vi "OE2011&OE2021_Configure Demodulator Reference.vi"(7 "OE2012&OE2022_Configure Demodulator Ref":T1={"Demodulator"=1, "Ref. Source"=0, "Arb Frequency"=1000.0, "Ref. Harmonic"=1, "Ref. Phase(degree)"=0.0, "Instrument Mode "=10, "A"=1000, "F1"=0, "B"=1000, "F2"=0} {"F2" items=["OSC1", "OSC2", "Demod MF1", "Demod MF2", "Demod MF3", "Demod MF4", "Demod MF5", "Demod MF6", "Demod MF7", "Demod MF8"]; "B" min=-10000 max=10000; "F1" items=["OSC1", "OSC2", "Demod MF1", "Demod MF2", "Demod MF3", "Demod MF4", "Demod MF5", "Demod MF6", "Demod MF7", "Demod MF8"]; "A" min=-10000 max=10000; "Instrument Mode" items=["OE2012"=10, "OE2022"=11]; "Ref. Phase(degree)" min=-180.0 max=180.0 format="%#.2g"; "Ref. Harmonic" min=1 max=32767; "Arb Frequency" min=1e-06 max=1002000.0 format="%#.3f"; "Ref. Source" items=["OSC1", "OSC2", "ManualFrequency", "FreqComb1", "FreqComb2", "FreqComb3", "FreqComb4"]; "Demodulator" items=["Demod1"=1, "Demod2"=2, "Demod3"=3, "Demod4"=4, "Demod5"=5, "Demod6"=6, "Demod7"=7, "Demod8"=8]}, 8 "Error in (no error)":errorcluster caption="error out（no error）", 9 "Remote Mode":u16(ring)=1 items=["USB", "RS232", "GPIB", "Ethernet"], 10 "Connection ID in":refnum<k5>, 11 "VISA resource name":refnum<visa-resource-name>) -> (0 "Error out":errorcluster caption="error out", 1 "Output String":string, 2 "Connection ID out":refnum<k5>, 3 "VISA resource  out":refnum<visa-resource-name>)   [LabVIEW 2011]
panel:
  out "Demod Channel":string
  # "E = A * Osc + B * Freq"
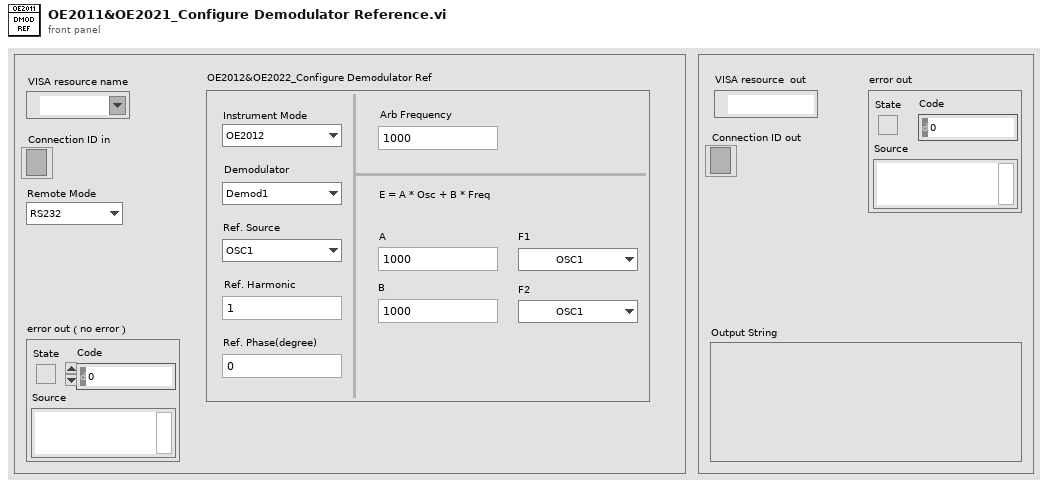
[diagram p1: front panel]
types:
  T1 = cluster{"Demodulator":u16, "Ref. Source":u16, "Arb Frequency":dbl, "Ref. Harmonic":u16, "Ref. Phase(degree)":dbl, "Instrument Mode ":u16, "A":i16, "F1":u16, "B":i16, "F2":u16}
  T2 = enum16{"ISRC", "IGND", "ICPL", "ILIN", "PHAS", "FMOD", "RSLP", "FREQ", "SWPT", "SLLM", "SULM", "SSLL", "SSLG", "STLM", "SWRM", "IRNG", "SENS", "RMOD", "OFLT", "OFSL", "SYNC", "DMOD", "HARM", "DARB", "SWVT", "SLVL", "SVLL", "SVUL", "SVSL", "SVSG", "SVTM", "SVRM", "RALL", "SNAP", "OUTP", "OAUX", "COUT", "CAUX", "COFP", "CEXP", "FPOP", "OEXP", "*IDN", "*RST", "OVLD", "INOV", "GNOV", "*PLL", "SSET", "RSET", "AGAN", "APHS", "ARSV", "ASCL", "EQCD", "EQCS", "SPED", "SRAT", "SLEN", "SSLE", "STRG", "SPRM", "STRD", "PAUS", "REST", "SPTS", "TRCA", "TEMP", "RSTU", "IHNZ", "DEQU", "SADD", "ARNG", "CSPE", "ISRCD", "IGNDD", "ICPLD", "ILIND", "PHASD", "FMODD", "RSLPD", "FREQD", "SWPTD", "SLLMD", "SULMD", "SSLLD", "SSLGD", "STLMD", "SWRMD", "SENSD", "RMODD", "OFLTD", "OFSLD", "SYNCD", "HARMD", "EQCDD", "EQCSD", "SNAPD", "OUTPD", "SWVTD", "SLVLD", "SVLLD", "SVULD", "SVSLD", "SVSGD", "SVTMD", "SVRMD", "SVDCD", "ARSVD", "AGAND", "APHSD", "ASCLD", "FPOPD", "CAUXD", "OEXPD", "SPEDD", "SRATD", "SLEND", "SSLED", "STRGD", "SPRMD", "STRDD", "PAUSD", "RESTD", "SPTSD", "TRCAD", "*IDND", "*RSTD", "INOVD", "GNOVD", "*PLLD", "SSETD", "RSETD", "RALLD"}
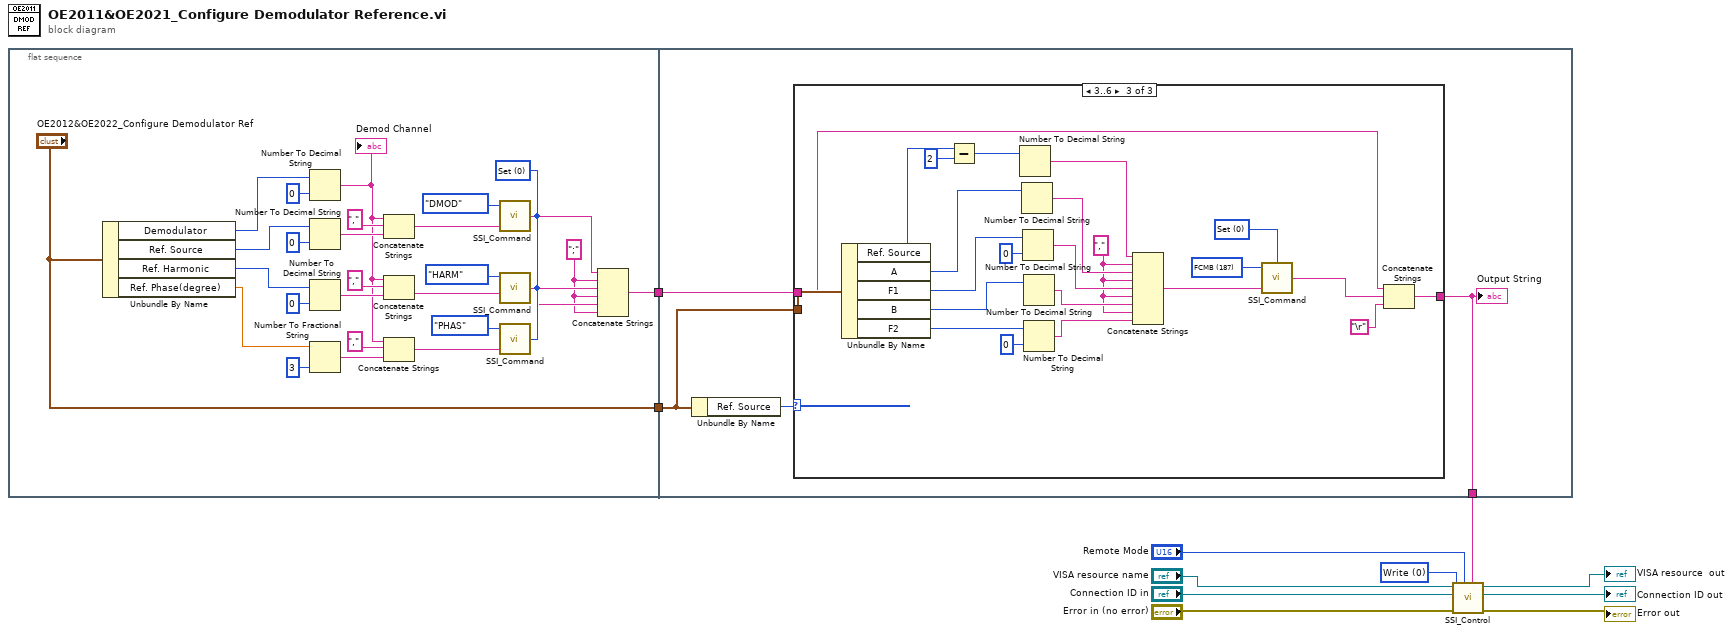
[diagram p0: block diagram]
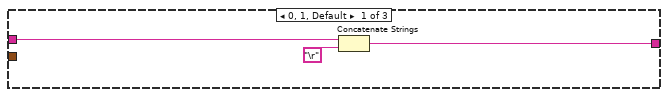
[diagram p2: hidden frame]
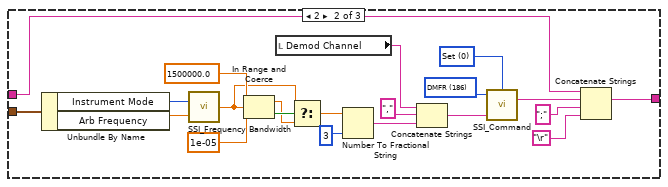
[diagram p3: hidden frame]
diagram:
  w9 = u16 0 items=["Write", "Read"] ("Control")
  n1 = flat-sequence {
    tunnel: [w13] -> w3
    tunnel: ["OE2012&OE2022_Configure Demodulator Ref"] -> w2
    tunnel: w3 -> [w41]
    tunnel: w2 -> [w42]
    tunnel: [w40] -> w1
    frame #0 {
      w23 = u16 0 items=["Set", "Query"] ("Opera")
      w18 = ";" ("字符串")
      n2 = Unbundle By Name("OE2012&OE2022_Configure Demodulator Ref") -> ("Demodulator"=w36:u16, "Ref. Source"=w31:u16, "Ref. Harmonic"=w28:u16, "Ref. Phase(degree)"=w20:dbl)
      n3 = Number To Decimal String(number=w36, width (-)=i16 0 ("精度(6)")) -> (decimal integer string=w14:string)
      "Demod Channel" <- w14
      n4 = Number To Decimal String(number=w31, width (-)=i16 0 ("精度(6)")) -> (decimal integer string=w32:string)
      n5 = Number To Decimal String(number=w28, width (-)=i16 0 ("精度(6)")) -> (decimal integer string=w29:string)
      n6 = Number To Fractional String(number=w20, precision (6)=i16 3 ("精度(6)")) -> (F-format string=w16:string)  [unwired: 2 in]
      n7 = Concatenate Strings(w14, "," ("字符串"), w32) -> (w35:string)
      n8 = Concatenate Strings(w14, "," ("字符串"), w29) -> (w34:string)
      n9 = Concatenate Strings(w14, "," ("字符串"), w16) -> (w15:string)
      n10 = call "SSI_Command.vi"("Opera"=w23, "Paramter"=w35, "Command Type"=T2."DMOD") -> ("Output string"=w27:string)  [unwired: 1 in]
      n11 = call "SSI_Command.vi"("Opera"=w23, "Paramter"=w34, "Command Type"=T2."HARM") -> ("Output string"=w26:string)  [unwired: 1 in]
      n12 = call "SSI_Command.vi"("Opera"=w23, "Paramter"=w15, "Command Type"=T2."PHAS") -> ("Output string"=w19:string)  [unwired: 1 in]
      n13 = Concatenate Strings(w27, w18, w26, w18, w19, w18) -> (w13:string)
    }
    frame #1 {
      n14 = Unbundle By Name(w42) -> ("Ref. Source"=w43:u16)
      n15 = case shown="3..6" w43 {
        tunnel: [w44 w60 w88] -> w40
        tunnel: w42 -> [_ w59 w90]
        tunnel: w41 -> [w46 w48 w87]
        frame 0, 1, Default {
          n16 = Concatenate Strings(w46, "\r") -> (w44:string)
        }
        frame 2 {
          w47 = u16 186 items=["ISRC", "IGND", "ICPL", "ILIN", "PHAS", "FMOD", "RSLP", "FREQ", "SWPT", "SLLM", "SULM", "SSLL", "SSLG", "STLM", "SWRM", "IRNG", "SENS", "RMOD", "OFLT", "OFSL", "SYNC", "DMOD", "HARM", "DARB", "SWVT", "SLVL", "SVLL", "SVUL", "SVSL", "SVSG", "SVTM", "SVRM", "RALL", "SNAP", "OUTP", "OAUX", "COUT", "CAUX", "COFP", "CEXP", "FPOP", "OEXP", "*IDN", "*RST", "OVLD", "INOV", "GNOV", "*PLL", "SSET", "RSET", "AGAN", "APHS", "ARSV", "ASCL", "EQCD", "EQCS", "SPED", "SRAT", "SLEN", "SSLE", "STRG", "SPRM", "STRD", "PAUS", "REST", "SPTS", "TRCA", "TEMP", "RSTU", "INHZ", "DEQU", "SADD", "ARNG", "CSPE", "ISRCD", "IGNDD", "ICPLD", "ILIND", "PHASD", "FMODD", "RSLPD", "FREQD", "SWPTD", "SLLMD", "SULMD", "SSLLD", "SSLGD", "STLMD", "SWRMD", "SENSD", "RMODD", "OFLTD", "OFSLD", "SYNCD", "HARMD", "EQCDD", "EQCSD", "SNAPD", "OUTPD", "SWVTD", "SLVLD", "SVLLD", "SVULD", "SVSLD", "SVSGD", "SVTMD", "SVRMD", "SVDCD", "ARSVD", "AGAND", "APHSD", "ASCLD", "FPOPD", "CAUXD", "OEXPD", "SPEDD", "SRATD", "SLEND", "SSLED", "STRGD", "SPRMD", "STRDD", "PAUSD", "RESTD", "SPTSD", "TRCAD", "*IDND", "*RSTD", "INOVD", "GNOVD", "*PLLD", "SSETD", "RSETD", "RALLD", "NIPA", "NSMA", "NGWA", "NMAC", "NMOD", "TRIG", "TRCB", "INHZD", "ISAMD", "IRAGD", "RRAGD", "SOFFD", "DMODD", "COUTD", "COFPD", "CEXPD", "ARNGD", "OAUXD", "TRIM", "SUITD", "SNHZD", "AOFSD", "RSRC", "FEXT", "FINT", "DSRC", "DARF", "DEAF", "DREF", "SSRC", "STTL", "SIGO", "SLVL", "SOFF", "SPHS", "TPHS", "SMOD", "MARF", "AMSR", "AMDP", "FMSR", "FMDV", "PMSR", "PMDV", "CHDC", "AUXV", "AFLT", "AOFP", "DSELD", "FEMSD", "SLVTD", "SLVBD", "DMFR", "FCMB", "SMFR"] ("Command Type")
          w49 = u16 0 items=["Set", "Query"] ("Opera")
          n17 = Unbundle By Name(w59) -> ("Instrument Mode"=w57:u16, "Arb Frequency"=w58:dbl)
          n18 = call "SSI_Frequency Bandwidth.vi"("Frequency"=w58, "Instrument Mode"=w57) -> ("Output"=w52:dbl)  [unwired: 1 in]
          n19 = In Range and Coerce(upper limit=1500000.0 ("上限"), x=w52, lower limit=1e-05 ("下限")) -> (coerced(x)=w55:dbl, In Range?=w56:bool)
          n20 = local read "Demod Channel"() -> (w50:string)
          n21 = Select(t=w52, s=w56, f=w55) -> (s? t:f=w51:dbl)
          n22 = Number To Fractional String(number=w51, precision (6)=i16 3 ("精度(6)")) -> (F-format string=w65:string)  [unwired: 2 in]
          n23 = Concatenate Strings(w50, "," ("字符串"), w65) -> (w67:string)
          n24 = call "SSI_Command.vi"("Opera"=w49, "Paramter"=w67, "Command Type"=w47) -> ("Output string"=w64:string)  [unwired: 1 in]
          n25 = Concatenate Strings(w48, w64, ";" ("字符串"), "\r") -> (w60:string)
        }
        frame 3..6 {
          w71 = u16 187 items=["ISRC", "IGND", "ICPL", "ILIN", "PHAS", "FMOD", "RSLP", "FREQ", "SWPT", "SLLM", "SULM", "SSLL", "SSLG", "STLM", "SWRM", "IRNG", "SENS", "RMOD", "OFLT", "OFSL", "SYNC", "DMOD", "HARM", "DARB", "SWVT", "SLVL", "SVLL", "SVUL", "SVSL", "SVSG", "SVTM", "SVRM", "RALL", "SNAP", "OUTP", "OAUX", "COUT", "CAUX", "COFP", "CEXP", "FPOP", "OEXP", "*IDN", "*RST", "OVLD", "INOV", "GNOV", "*PLL", "SSET", "RSET", "AGAN", "APHS", "ARSV", "ASCL", "EQCD", "EQCS", "SPED", "SRAT", "SLEN", "SSLE", "STRG", "SPRM", "STRD", "PAUS", "REST", "SPTS", "TRCA", "TEMP", "RSTU", "INHZ", "DEQU", "SADD", "ARNG", "CSPE", "ISRCD", "IGNDD", "ICPLD", "ILIND", "PHASD", "FMODD", "RSLPD", "FREQD", "SWPTD", "SLLMD", "SULMD", "SSLLD", "SSLGD", "STLMD", "SWRMD", "SENSD", "RMODD", "OFLTD", "OFSLD", "SYNCD", "HARMD", "EQCDD", "EQCSD", "SNAPD", "OUTPD", "SWVTD", "SLVLD", "SVLLD", "SVULD", "SVSLD", "SVSGD", "SVTMD", "SVRMD", "SVDCD", "ARSVD", "AGAND", "APHSD", "ASCLD", "FPOPD", "CAUXD", "OEXPD", "SPEDD", "SRATD", "SLEND", "SSLED", "STRGD", "SPRMD", "STRDD", "PAUSD", "RESTD", "SPTSD", "TRCAD", "*IDND", "*RSTD", "INOVD", "GNOVD", "*PLLD", "SSETD", "RSETD", "RALLD", "NIPA", "NSMA", "NGWA", "NMAC", "NMOD", "TRIG", "TRCB", "INHZD", "ISAMD", "IRAGD", "RRAGD", "SOFFD", "DMODD", "COUTD", "COFPD", "CEXPD", "ARNGD", "OAUXD", "TRIM", "SUITD", "SNHZD", "AOFSD", "RSRC", "FEXT", "FINT", "DSRC", "DARF", "DEAF", "DREF", "SSRC", "STTL", "SIGO", "SLVL", "SOFF", "SPHS", "TPHS", "SMOD", "MARF", "AMSR", "AMDP", "FMSR", "FMDV", "PMSR", "PMDV", "CHDC", "AUXV", "AFLT", "AOFP", "DSELD", "FEMSD", "SLVTD", "SLVBD", "DMFR", "FCMB", "SMFR"] ("Command Type")
          w78 = "," ("字符串")
          w75 = u16 0 items=["Set", "Query"] ("Opera")
          n26 = Unbundle By Name(w90) -> ("Ref. Source"=w70:u16, "A"=w86:i16, "F1"=w83:u16, "B"=w85:i16, "F2"=w73:u16)
          n27 = Subtract(x=w70, y=u16 2) -> (x-y=w68:u16)
          n28 = Number To Decimal String(number=w68) -> (decimal integer string=w72:string)  [unwired: 1 in]
          n29 = Number To Decimal String(number=w86) -> (decimal integer string=w81:string)  [unwired: 1 in]
          n30 = Number To Decimal String(number=w83, width (-)=i16 0 ("精度(6)")) -> (decimal integer string=w80:string)
          n31 = Number To Decimal String(number=w85) -> (decimal integer string=w79:string)  [unwired: 1 in]
          n32 = Number To Decimal String(number=w73, width (-)=i16 0 ("精度(6)")) -> (decimal integer string=w77:string)
          n33 = Concatenate Strings(w72, w78, w81, w78, w80, w78, w79, w78, w77) -> (w89:string)
          n34 = call "SSI_Command.vi"("Opera"=w75, "Paramter"=w89, "Command Type"=w71) -> ("Output string"=w76:string)  [unwired: 1 in]
          n35 = Concatenate Strings(w87, w76, "\r") -> (w88:string)
        }
      }
      "Output String" <- w40
    }
  }
  n36 = call "SSI_Control.vi"("Write Buffer"=w1, "Remote Mode"="Remote Mode", "Error in (no error)"="Error in (no error)", "Control"=w9, "Connection ID in"="Connection ID in", "VISA resource name"="VISA resource name") -> ("Error out"=→"Error out":errorcluster, "Connection ID out"=→"Connection ID out":refnum<k5>, "VISA resource  out"=→"VISA resource  out":refnum<visa-resource-name>)  [unwired: 2 in, 1 out]
